vi "USB-IRSND.vi"(2 "error in (no error)":errorcluster caption="Fehler (Eingang, kein Fehler)", 3 "irmp_data":T2={"protocol"=11, " address"=135, " command"=104, " flags"=1} {"address" format="%04x"; "flags" format="%02x"; "command" format="%04x"; "protocol" items=["no protocol", "SIRCS (Sony)", "NEC (NEC, Pioneer, JVC, Toshiba, NoName...)", "SAMSUNG", "MATSUSHITA", "KASEIKYO (Panasonic)", "RECS80 (Philips, Thomson, Nordmende, Telefunken, Saba)", "RC5 (Philips, ...)", "DENON (Denon, Sharp)", "RC6 (Philips, ...)", "SAMSUNG32 (Samsung)", "APPLE", "RECS80EXT (Philips, Technisat, Thomson, Nordmende, Telefunken, Saba)", "NUBERT", "BANG_OLUFSON", "GRUNDIG", "NOKIA", "SIEMENS", "FDC", "RCCAR", "JVC", "RC6A (Kathrein, XBox)", "NIKON", "RUWIDO", "IR60", "KATHREIN", "NETBOX", "NEC16", "NEC42", "LEGO", "THOMSON", "BOSE"]}, 4 "IRSND USB Device":refnum<visa-resource-name>) -> (0 "error out":errorcluster caption="Fehler (Ausgang)")   [LabVIEW 2009]
panel:
  out "irmp_data (lb / hb)":T1={"protocol"=11, " address LB"=135, " address HB"=135, " command LB"=104, " command HB"=104, " flags"=1} {"command LB" format="%02x"; "address HB" format="%02x"; "flags" format="%02x"; "command HB" format="%02x"; "address LB" format="%02x"; "protocol" items=["no protocol", "SIRCS (Sony)", "NEC (NEC, Pioneer, JVC, Toshiba, NoName...)", "SAMSUNG", "MATSUSHITA", "KASEIKYO (Panasonic)", "RECS80 (Philips, Thomson, Nordmende, Telefunken, Saba)", "RC5 (Philips, ...)", "DENON (Denon, Sharp)", "RC6 (Philips, ...)", "SAMSUNG32 (Samsung)", "APPLE", "RECS80EXT (Philips, Technisat, Thomson, Nordmende, Telefunken, Saba)", "NUBERT", "BANG_OLUFSON", "GRUNDIG", "NOKIA", "SIEMENS", "FDC", "RCCAR", "JVC", "RC6A (Kathrein, XBox)", "NIKON", "RUWIDO", "IR60", "KATHREIN", "NETBOX", "NEC16", "NEC42", "LEGO", "THOMSON", "BOSE"]}
  # "Correction for LabVIEWs big endian byte order..."
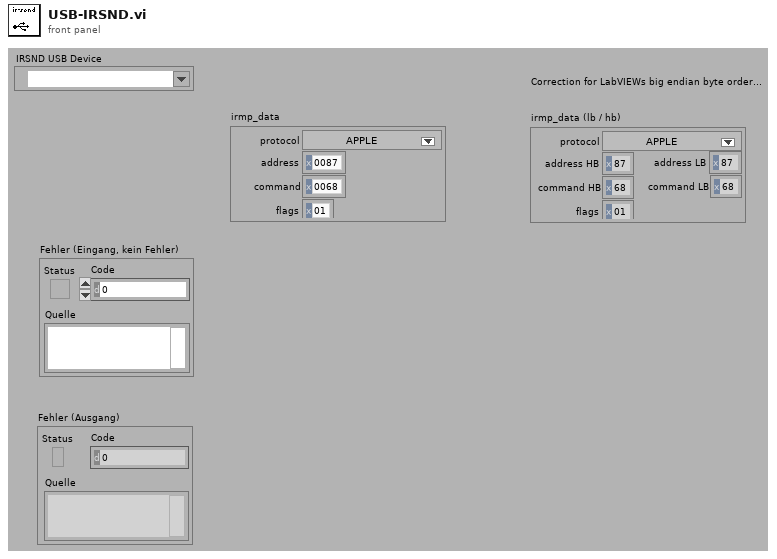
[diagram p1: front panel]
types:
  T1 = cluster{"protocol":u8, " address LB":u8, " address HB":u8, " command LB":u8, " command HB":u8, " flags":u8}
  T2 = cluster{"protocol":u8, " address":u16, " command":u16, " flags":u8}
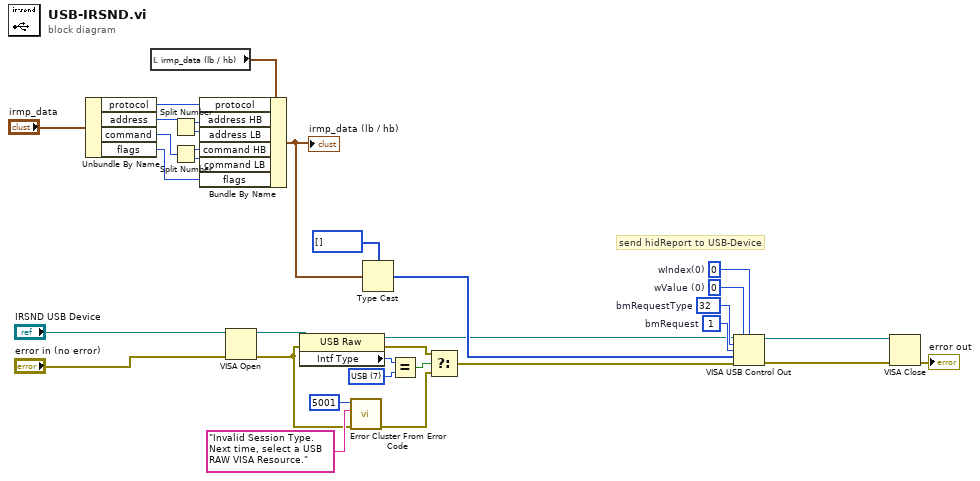
[diagram p0: block diagram]
diagram:
  w16 = i16 1  # bmRequest
  w19 = i16 32  # bmRequestType
  w15 = u16 0  # wValue (0)
  w14 = u16 0  # wIndex(0)
  w31 = u16 7 items=["GPIB"=1, "VXI"=2, "GPIB-VXI"=3, "Serial"=4, "PXI"=5, "TCPIP"=6, "USB"=7] ("Interface Information:Interface Type")
  # "send hidReport to USB-Device"
  n1 = Unbundle By Name("irmp_data") -> ("protocol"=w10:u8, "address"=w7:u16, "command"=w3:u16, "flags"=w9:u8)
  n2 = local read "irmp_data (lb / hb)"() -> (w1:T1)
  n3 = Split Number(x=w7) -> (hi(x)=w8:u8, lo(x)=w6:u8)
  n4 = Split Number(x=w3) -> (hi(x)=w5:u8, lo(x)=w4:u8)
  n5 = Bundle By Name(cluster=w1, "protocol"=w10, "address HB"=w8, "address LB"=w6, "command HB"=w5, "command LB"=w4, "flags"=w9) -> (w2:T1)
  "irmp_data (lb / hb)" <- w2
  n6 = VISA Open(error in (no error)="error in (no error)", VISA resource name="IRSND USB Device") -> (VISA resource name=w12:refnum<visa-resource-name>, error out=w26:errorcluster)  [unwired: 3 in]
  n7 = property class="USB Raw"(reference=w12, error in=w26) -> (reference out=w13:refnum<visa-resource-name>, error out=w30:errorcluster, "Intf Type"=w32:u16)
  n8 = call <vilib>:"Error Cluster From Error Code.vi"("error in (no error)"=w26, "error message (\"\")"="Invalid Session Type.  Next time, select a USB RAW VISA Resource." ("error message (\"\")"), "error code (0)"=5001) -> ("error out"=w25:errorcluster)  [unwired: 1 in, 5 out]
  n9 = Type Cast(type=u8[] [], x=w2) -> (*(type *) &x=w18:u8[])
  n10 = Equal?(x=w32, y=w31) -> (x = y?=w29:bool)
  n11 = Select(t=w30, s=w29, f=w25) -> (s? t:f=w17:errorcluster)
  n12 = VISA USB Control Out(0:w13, 1:w15, 2:w14, 5:w19, 7:w16, 9:w18, 11:w17) -> (4:w22:refnum<visa-resource-name>, 15:w21:errorcluster)
  n13 = VISA Close(VISA resource name=w22, error in (no error)=w21) -> (error out=→"error out":errorcluster)
